vi "Filtrado y discrim. de datos.vi"(6 "Frecuencia de muestreo":dbl, 9 "dt RMS":dbl, 10 "Arreglo de datos leidos del archivo":sgl[](array[numeric]), 11 "Parámetros del acelerómetro":dbl) -> (3 "Máximo por ejes":dbl)   [LabVIEW 2015]
uses:
  <vilib>/Analysis/3filter.llb/Filter Passband Type.ctl
  <vilib>/Analysis/5stat.llb/RMS (DBL).vi
  <vilib>/Analysis/3filter.llb/Butterworth Filter (DBL).vi
  <vilib>/measure/madcrms.llb/Basic Averaged DC-RMS for 1 Chan.vi
  <vilib>/Analysis/NI_AALPro.lvlib
  <vilib>/measure/NI_MAPro.lvlib
  <vilib>/Analysis/NI_AALBase.lvlib
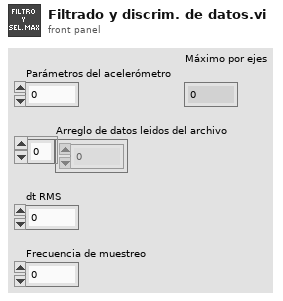
[diagram p1: front panel]
types:
  T1 = typedef "NI_AALBase.lvlib/Filter Passband Type.ctl" = enum32{"Lowpass", "Highpass", "Bandpass", "Bandstop"}
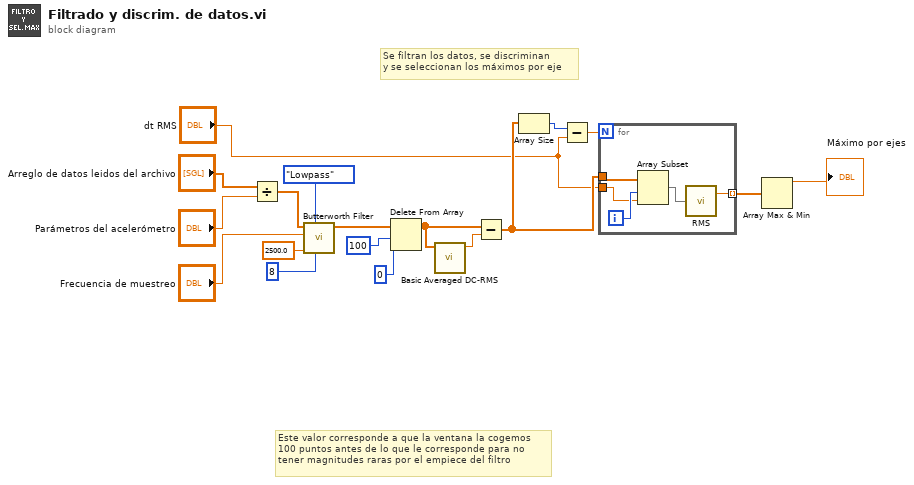
[diagram p0: block diagram]
diagram:
  # "Se filtran los datos, se discriminan\ny se seleccionan los máximos por eje"
  # "Este valor corresponde a que la ventana la cogemos\n100 puntos antes de lo que le corresponde para no \ntener magnitudes raras por el empiece del filtro"
  n1 = Divide(x="Arreglo de datos leidos del archivo", y="Parámetros del acelerómetro") -> (x/y=w9:dbl[])
  n2 = call-poly <vilib>:"Butterworth Filter.vi"("order"=8, "filter type"=Filter_Passband_Type."Lowpass", "low cutoff freq: fl"=2500.0, "sampling freq: fs"="Frecuencia de muestreo", "X"=w9) -> ("Filtered X"=w10:dbl[])  [unwired: 3 in, 1 out]
  n3 = Delete From Array(array=w10, length=100, index=0) -> (array with subset deleted=w11:dbl[])  [unwired: 1 out]
  n4 = call-poly <vilib>:"Basic Averaged DC-RMS.vi"("signal in"=w11) -> ("DC value"=w6:dbl)  [unwired: 4 in, 6 out]
  n5 = Subtract(x=w11, y=w6) -> (x-y=w18:dbl[])
  n6 = Array Size(array=w18) -> (size(s)=w3:i32)
  n7 = Subtract(x=w3, y="dt RMS") -> (x-y=w2:dbl)
  n8 = for {
    N: w2 -> [_]
    tunnel: "dt RMS" -> [w20]
    tunnel: [w23] -> w5 mode=indexing
    tunnel: w18 -> [w22]
    i -> [w21]
    n9 = Array Subset(array=w22, index=w21, length=w20) -> (w19:dbl[])
    n10 = call-poly <vilib>:"RMS.vi"("X"=w19) -> ("rms value"=w23:dbl)  [unwired: 1 out]
  }
  n11 = Array Max & Min(array=w5) -> (max value=→"Máximo por ejes":dbl)  [unwired: 3 out]
